vi "Main.vi"() -> ()   [LabVIEW 2017]
uses:
  <vilib>/rvi/Analysis/control/PID/Typedef/niFpgaPID_PIGains.ctl
  modulationConfig.ctl
  FPGA/contState.ctl
  <vilib>/NI/PowerElectronicsControl/ScaleAndLimit/Interface/Configuration.ctl
  <vilib>/NI/PowerElectronicsControl/BufferLogging/BufferConfig.ctl
  TuningParameters.ctl
  <instrlib>/_niInstr/FIFO Register Bus/v1/Host/niInstr FIFO Register Bus v1 Host.lvclass
  C:/Program Files (x86)/National Instruments/LabVIEW 2017/instr.lib/_niInstr/Instruction Framework/v1/Host/Instruction Target/niInstr Instruction Target v1 Host.lvclass
  <vilib>/FPGAPlugInAG/sbRIO-9607/niLvFpga_Open_sbRIO-9607.vi
  <vilib>/rvi/interface/common/dynamic/niFpgaDynamicAddResources.vi
  <vilib>/FPGAPlugInAG/Dynamic/niLvFpga_Reset_Dynamic.vi
  <vilib>/FPGAPlugInAG/Dynamic/niLvFpga_Run_Dynamic.vi
  <vilib>/Utility/error.llb/Error Cluster From Error Code.vi
  <vilib>/RVI Host/nirviSupport.llb/nirviErrorClusterFromErrorCode.vi
  <vilib>/rvi/errors/niLvFpgaAdjustHostInterfaceError.vi
  <vilib>/NI/PowerElectronicsControl/WaveformAcq/RT/ReadInterleaved.vi
  <vilib>/FPGAPlugInAG/Dynamic/niLvFpga_Close_Dynamic.vi
  <vilib>/rvi/interface/nirviOpenFPGA/nirviOpenFPGA.xnode
  FPGA Bitfiles/BuckBoost_FPGATarget_Firmware_5T++5BilX3c.lvbitx
  FPGA/Firmware.vi
  <vilib>/rvi/interface/nirviMethod/nirviMethod.xnode
  <vilib>/rvi/interface/nirviReadWriteControl/nirviReadWriteControl.xnode
  <vilib>/rvi/interface/nirviCloseFPGA/nirviCloseFPGA.xnode
  <vilib>/NI/PowerElectronicsControl/ScaleAndLimit/Interface/ScaleAndLimitInterface.lvlib
  <instrlib>/_niInstr/Instruction Framework/v1/Host/Subsystem Map/niInstr Subsystem Map v1 Host.lvclass
  <vilib>/NI/PowerElectronicsControl/WaveformAcq/RT/WaveformTask.lvclass
  <vilib>/NI/PowerElectronicsControl/BufferLogging/BufferLogging.lvlib
  <vilib>/rvi/interface/nirviMethod/StockFPGA_InlinedMethodWaitForSingleIRQ.vi
  <vilib>/FPGAPlugInAG/Dynamic/niLvFpga_WaitOnIrq_Dynamic.vi
  <vilib>/rvi/interface/Simulation/niFpgaSimulationCallBeginRW.vi
  <vilib>/FPGAPlugInAG/Dynamic/niLvFpga_AcknowledgeIrq_Dynamic.vi
  NiFpgaLv.dll
  BuckBoostInterface.lvlib
  FPGA/BuckBoost.lvlib
panel:
  in  "Tab Control":enum32{"Monitoring", "BuckBoost"}(tab)=enum."BuckBoost"
  out "SimultaneousAI":sgl[](array[numeric])=[-0.17586, 0.33218002, -0.12701, 12.40282, 40.089428, 0.0, 0.0, 0.0, -0.0, 0.0, 0.0, 0.0, 0.0, 0.0, 0.0, 0.0]
  out "snapshot":waveform(sgl)[](graph)=[{"t0"=timestamp(0 s since 1904-01-01), "dt"=1e-05, "Y"=array[10000 elements]}, {"t0"=timestamp(0 s since 1904-01-01), "dt"=1e-05, "Y"=array[10000 elements]}, {"t0"=timestamp(0 s since 1904-01-01), "dt"=1e-05, "Y"=array[10000 elements]}, {"t0"=timestamp(0 s since 1904-01-01), "dt"=1e-05, "Y"=array[10000 elements]}, {"t0"=timestamp(0 s since 1904-01-01), "dt"=1e-05, "Y"=array[10000 elements]}, {"t0"=timestamp(0 s since 1904-01-01), "dt"=1e-05, "Y"=array[10000 elements]}, {"t0"=timestamp(0 s since 1904-01-01), "dt"=1e-05, "Y"=array[10000 elements]}, {"t0"=timestamp(0 s since 1904-01-01), "dt"=1e-05, "Y"=array[10000 elements]}, {"t0"=timestamp(0 s since 1904-01-01), "dt"=1e-05, "Y"=array[10000 elements]}, {"t0"=timestamp(0 s since 1904-01-01), "dt"=1e-05, "Y"=array[10000 elements]}, {"t0"=timestamp(0 s since 1904-01-01), "dt"=1e-05, "Y"=array[10000 elements]}, {"t0"=timestamp(0 s since 1904-01-01), "dt"=1e-05, "Y"=array[10000 elements]}, {"t0"=timestamp(0 s since 1904-01-01), "dt"=1e-05, "Y"=array[10000 elements]}, {"t0"=timestamp(0 s since 1904-01-01), "dt"=1e-05, "Y"=array[10000 elements]}, {"t0"=timestamp(0 s since 1904-01-01), "dt"=1e-05, "Y"=array[10000 elements]}, {"t0"=timestamp(0 s since 1904-01-01), "dt"=1e-05, "Y"=array[10000 elements]}, {"t0"=timestamp(0 s since 1904-01-01), "dt"=1e-05, "Y"=array[10000 elements]}, {"t0"=timestamp(0 s since 1904-01-01), "dt"=1e-05, "Y"=array[10000 elements]}]
  in  "Update Time (s)":dbl=2.0 caption="Time Target (s)" min=1.0
  in  "stop":bool
  in  "clearLimits":bool
  out "SimultaneousAILoopRate":u32=800
  out "Limits":string="Zero limits reached"
  in  "ManualTrigger":bool
  out "TotalCurrent":sgl
  out "Enabled":u8=7 format="%.0x"
  in  "I_setpt":sgl=10.0
  out "error":sgl[](array[numeric])=[0.17586, -0.33218002, 0.12701, 0.0]
  in  "Enable":bool=TRUE
  in  "pertAmp":sgl=1.0
  in  "pertFreq":sgl=10.0
  in  "controlFreq":sgl=50000.0
  in  "rampRate":sgl=0.0001
  in  "state":T1=enum."normal"
  in  "gains":T2={"proportional gain"=0.1, "integral gain"=1e-05} {"proportional gain" step=0.125}
  in  "modulationConfig":T3={"SwitchingSpeed"=5000.0, "Deadband"=1e-07, "modulationRate"=40000000.0}
  in  "manualInput":sgl
  in  "UpdateConfig":bool
  out "actualBuckBoostRate":u32=800
  # "CAREFUL"
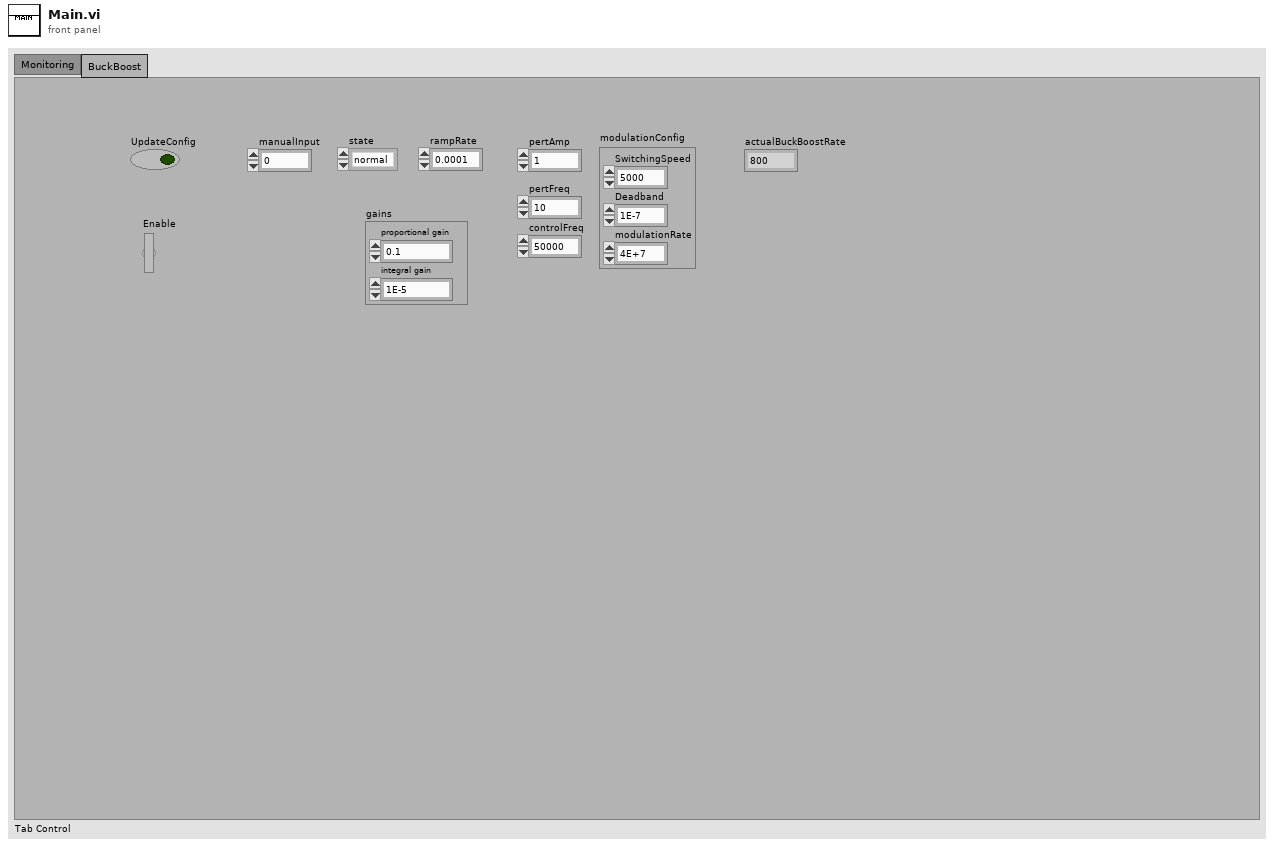
[diagram p1: front panel]
types:
  T1 = typedef "BuckBoost.lvlib/contState.ctl" = enum16{"disabled", "manual", "normal", "perturb"}
  T2 = typedef "niFpgaPID_PIGains.ctl" = cluster{"proportional gain":sgl, "integral gain":sgl}
  T3 = typedef "BuckBoostInterface.lvlib/modulationConfig.ctl" = cluster{"SwitchingSpeed":dbl, "Deadband":dbl, "modulationRate":dbl}
  T4 = typedef "BuckBoostInterface.lvlib/TuningParameters.ctl" = cluster{"gains":T2, "manualInput":sgl, "rampRate":sgl, "pertAmp":sgl, "pertFreq":sgl, "controlFreq":sgl, "state":T1}
  T5 = typedef "BufferLogging.lvlib/BufferConfig.ctl" = cluster{"Channels":string[], "pretriggerTime_sec":dbl, "posttriggerTime_sec":dbl, "BlockSizePerChannel":i32, "SampleRate_Hz":dbl, "decimation factor":i32, "logDirectory":string, "logPrefix":string, "max files":i32}
  T6 = typedef "ScaleAndLimitInterface.lvlib/Configuration.ctl" = cluster{"Name":string, "M":dbl, "B":i16, "HighLimit":dbl, "LowLimit":dbl, "LimitsEnabled":bool}
  T7 = typedef "BufferLogging.lvlib/Buffers.ctl" = cluster{"Channels":string[], "PosttriggerBuffer":refnum<queue>, "PretriggerBuffer":refnum<queue>, "BlockSizePerChannel":i32, " logging semaphore":T8, "Log refnum":refnum<k34>, "snapshotBuffer":refnum<data-value>, "logDirectory":path, "logPrefix":string, "decimation factor":i32, "max files":i32, "SampleRate":dbl}
  T8 = typedef "Semaphore RefNum" = refnum<k1>
  T9 = typedef "BuckBoostInterface.lvlib/Interface.ctl" = cluster{"instruction target":refnum<class "niInstr Instruction Target v1 Host.lvclass">, "BuckBoostContext":refnum<class "niInstr Instruction Framework Context v1 Host.lvclass">}
  T10 = typedef "ScaleAndLimitInterface.lvlib/Interface.ctl" = cluster{"instruction target":refnum<class "niInstr Instruction Target v1 Host.lvclass">, "ScalingAndLimitsContext":refnum<class "niInstr Instruction Framework Context v1 Host.lvclass">, "Configuration":T6[]}
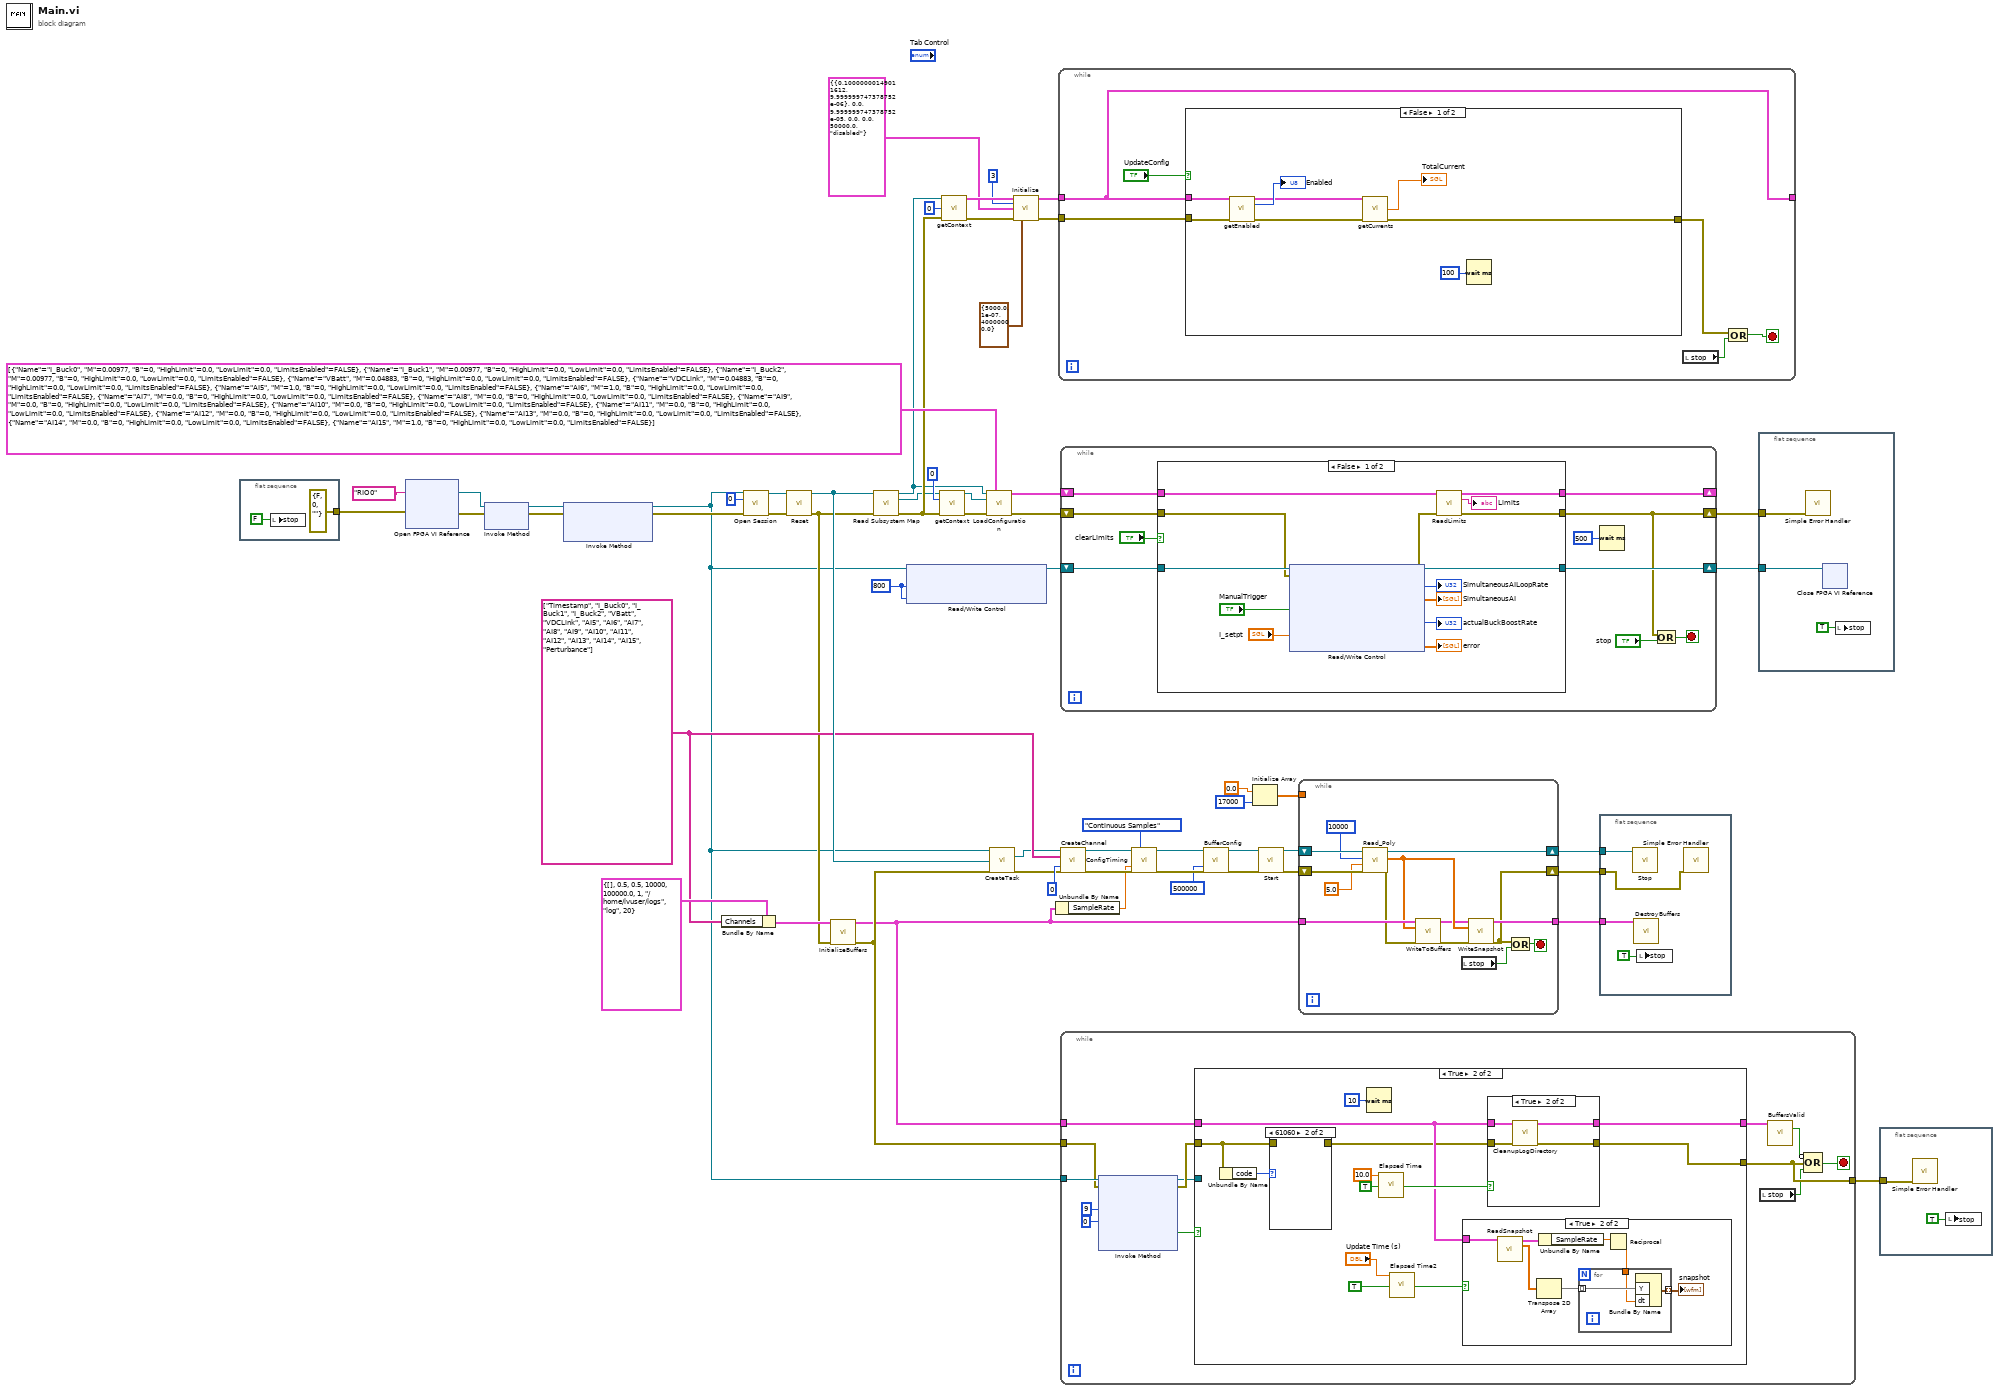
[diagram p0: block diagram]
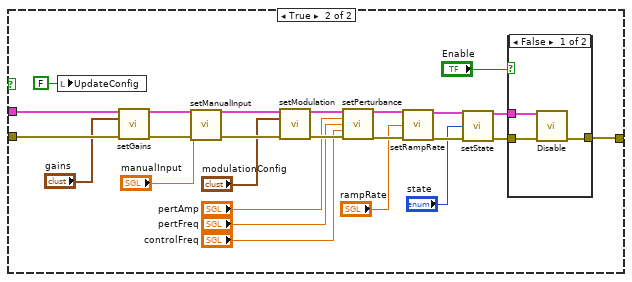
[diagram p2: hidden frame]
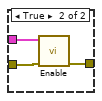
[diagram p3: hidden frame]
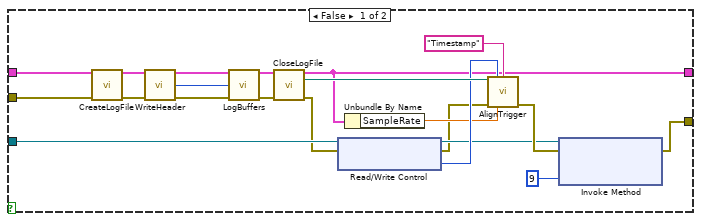
[diagram p4: hidden frame]
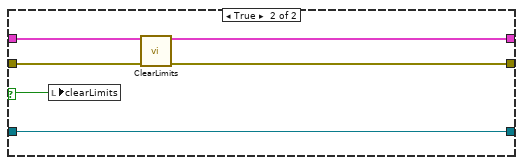
[diagram p8: hidden frame]
diagram:
  w13 = u32 800 ("desiredBuckBoostRate")
  w49 = string[] ["Timestamp", "I_Buck0", "I_Buck1", "I_Buck2", "VBatt", "VDCLink", "AI5", "AI6", "AI7", "AI8", "AI9", "AI10", "AI11", "AI12", "AI13", "AI14", "AI15", "Perturbance"] ("Chan Name Array")
  n1 = flat-sequence {
    tunnel: [errorcluster {"status"=FALSE, "code"=0, "source"=""} ("error in")] -> w46
    frame #0 {
      n2 = local write "stop"(FALSE ("stop")) -> ()
    }
  }
  n3 = xnode "Open FPGA VI Reference"("error in"=w46, "resource name"=tag "RIO0") -> ("FPGA VI Reference Out"=w6:refnum<k20>, "error out"=w5:errorcluster)
  n4 = xnode "Invoke Method"("FPGA VI Reference In"=w6, "error in"=w5) -> ("FPGA VI Reference Out"=w4:refnum<k20>, "error out"=w3:errorcluster)
  n5 = xnode "Invoke Method"("FPGA VI Reference In"=w4, "error in"=w3) -> ("FPGA VI Reference Out"=w1:refnum<k20>, "error out"=w2:errorcluster)  [unwired: 1 in]
  n6 = Bundle By Name(cluster=T5 {"Channels"=[], "pretriggerTime_sec"=0.5, "posttriggerTime_sec"=0.5, "BlockSizePerChannel"=10000, "SampleRate_Hz"=100000.0, "decimation factor"=1, "logDirectory"="/home/lvuser/logs", "logPrefix"="log", "max files"=20} ("BufferConfig"), "Channels"=w49) -> (w48:T5)
  n7 = call <instrlib>:"Open Session.vi"("fpga ref"=w1, "bus instance"=u32 0, "error in"=w2) -> ("session out"=w53:refnum<class "niInstr FIFO Register Bus v1 Host.lvclass">, "error out"=w54:errorcluster)  [unwired: 11 in]
  n8 = call-dynamic "Reset.vi"("session in"=w53, "error in"=w54) -> ("session out"=w51:refnum<class "niInstr FIFO Register Bus v1 Host.lvclass">, "error out"=w47:errorcluster)  [unwired: 12 in]
  n9 = call <vilib>:"InitializeBuffers.vi"("BufferConfig"=w48, "error in (no error)"=w47) -> ("Buffers"=w43:T7, "error out"=w44:errorcluster)  [unwired: 12 in]
  n10 = call <instrlib>:"Read Subsystem Map.vi"("instruction target in"=w51, "error in"=w47) -> ("instruction target out"=w9:refnum<class "niInstr FIFO Register Bus v1 Host.lvclass">, "subsystem map"=w8:refnum<class "niInstr Subsystem Map v1 Host.lvclass">, "error out"=w11:errorcluster)  [unwired: 11 in]
  n11 = xnode "Read/Write Control"("FPGA VI Reference In"=w1, "desiredBuckBoostRate"=w13, "desiredSimultaneousAILoopRate"=w13) -> ("FPGA VI Reference Out"=w14:refnum<k20>)  [unwired: 1 in, 1 out]
  n12 = call <vilib>:"getContext.vi"("subsystemMap"=w8, "instance"=u8 0, "error in"=w11) -> ("ScalingAndLimitsContext"=w10:refnum<class "niInstr Instruction Framework Context v1 Host.lvclass">, "error out"=w60:errorcluster)  [unwired: 11 in]
  n13 = call <vilib>:"getContext.vi"("instruction target in"=w9, "instance"=u8 0, "error in"=w11) -> ("Interface"=w20:T9, "error out"=w19:errorcluster)  [unwired: 11 in]
  n14 = call <vilib>:"LoadConfiguration.vi"("instruction target in"=w9, "Configuration"=T6[] [{"Name"="I_Buck0", "M"=0.00977, "B"=0, "HighLimit"=0.0, "LowLimit"=0.0, "LimitsEnabled"=FALSE}, {"Name"="I_Buck1", "M"=0.00977, "B"=0, "HighLimit"=0.0, "LowLimit"=0.0, "LimitsEnabled"=FALSE}, {"Name"="I_Buck2", "M"=0.00977, "B"=0, "HighLimit"=0.0, "LowLimit"=0.0, "LimitsEnabled"=FALSE}, {"Name"="VBatt", "M"=0.04883, "B"=0, "HighLimit"=0.0, "LowLimit"=0.0, "LimitsEnabled"=FALSE}, {"Name"="VDCLink", "M"=0.04883, "B"=0, "HighLimit"=0.0, "LowLimit"=0.0, "LimitsEnabled"=FALSE}, {"Name"="AI5", "M"=1.0, "B"=0, "HighLimit"=0.0, "LowLimit"=0.0, "LimitsEnabled"=FALSE}, {"Name"="AI6", "M"=1.0, "B"=0, "HighLimit"=0.0, "LowLimit"=0.0, "LimitsEnabled"=FALSE}, {"Name"="AI7", "M"=0.0, "B"=0, "HighLimit"=0.0, "LowLimit"=0.0, "LimitsEnabled"=FALSE}, {"Name"="AI8", "M"=0.0, "B"=0, "HighLimit"=0.0, "LowLimit"=0.0, "LimitsEnabled"=FALSE}, {"Name"="AI9", "M"=0.0, "B"=0, "HighLimit"=0.0, "LowLimit"=0.0, "LimitsEnabled"=FALSE}, {"Name"="AI10", "M"=0.0, "B"=0, "HighLimit"=0.0, "LowLimit"=0.0, "LimitsEnabled"=FALSE}, {"Name"="AI11", "M"=0.0, "B"=0, "HighLimit"=0.0, "LowLimit"=0.0, "LimitsEnabled"=FALSE}, {"Name"="AI12", "M"=0.0, "B"=0, "HighLimit"=0.0, "LowLimit"=0.0, "LimitsEnabled"=FALSE}, {"Name"="AI13", "M"=0.0, "B"=0, "HighLimit"=0.0, "LowLimit"=0.0, "LimitsEnabled"=FALSE}, {"Name"="AI14", "M"=0.0, "B"=0, "HighLimit"=0.0, "LowLimit"=0.0, "LimitsEnabled"=FALSE}, {"Name"="AI15", "M"=1.0, "B"=0, "HighLimit"=0.0, "LowLimit"=0.0, "LimitsEnabled"=FALSE}], "ScalingAndLimitsContext"=w10, "error in (no error)"=w60) -> ("Interface"=w57:T10, "error out"=w56:errorcluster)  [unwired: 10 in]
  n15 = call <vilib>:"CreateTask.vi"("FPGA Ref in"=w1, "session in"=w51, "error in"=w44) -> ("Task out"=w30:refnum<class "WaveformTask.lvclass">, "error out"=w29:errorcluster)  [unwired: 9 in, 2 out]
  n16 = call "Initialize.vi"("Interface in"=w20, "numOfInterleaves"=u8 3, "TuningParameters"=T4 {"gains"={"proportional gain"=0.1, "integral gain"=1e-05}, "manualInput"=0.0, "rampRate"=0.0001, "pertAmp"=0.0, "pertFreq"=0.0, "controlFreq"=50000.0, "state"=enum."disabled"}, "error in"=w19, "modulationConfig"=T3 {"SwitchingSpeed"=5000.0, "Deadband"=1e-07, "modulationRate"=40000000.0}) -> ("Interface out"=w16:T9, "error out"=w15:errorcluster)  [unwired: 9 in]
  n17 = Unbundle By Name(w43) -> ("SampleRate"=w26:dbl)
  n18 = while {
    tunnel: w16 -> [w67]
    tunnel: w15 -> [w68]
    tunnel: [w67] -> _
    stop <- w65 stop-if-true
    n19 = case shown="False" "UpdateConfig" {
      tunnel: w68 -> [w72 w100]
      tunnel: w67 -> [w73 w101]
      tunnel: [w69 w77] -> w64
      frame False {
        n20 = call "getEnabled.vi"("Interface in"=w73, "error in (no error)"=w72) -> ("Interface out"=w70:T9, "Enabled"=→"Enabled":u8, "error out"=w71:errorcluster)  [unwired: 11 in]
        n21 = call "getCurrents.vi"("Interface in"=w70, "error in (no error)"=w71) -> ("TotalCurrent"=→"TotalCurrent":sgl, "error out"=w69:errorcluster)  [unwired: 10 in, 2 out]
        n22 = Wait (ms)(milliseconds to wait=u32 100) -> ()  [unwired: 1 out]
      }
      frame True {
        n23 = local write "UpdateConfig"(FALSE ("UpdateConfig")) -> ()
        n24 = call "setGains.vi"("Interface in"=w101, "gains"="gains", "error in (no error)"=w100) -> ("Interface out"=w98:T9, "error out"=w99:errorcluster)  [unwired: 11 in]
        n25 = call "setManualInput.vi"("Interface in"=w98, "manualInput"="manualInput", "error in (no error)"=w99) -> ("Interface out"=w97:T9, "error out"=w96:errorcluster)  [unwired: 11 in]
        n26 = call "setModulation.vi"("Interface in"=w97, "modulationConfig"="modulationConfig", "error in (no error)"=w96) -> ("Interface out"=w94:T9, "error out"=w95:errorcluster)  [unwired: 11 in]
        n27 = call "setPerturbance.vi"("Interface in"=w94, "pertAmp"="pertAmp", "pertFreq"="pertFreq", "controlFreq"="controlFreq", "error in (no error)"=w95) -> ("Interface out"=w93:T9, "error out"=w90:errorcluster)  [unwired: 9 in]
        n28 = call "setRampRate.vi"("Interface in"=w93, "rampRate"="rampRate", "error in (no error)"=w90) -> ("Interface out"=w92:T9, "error out"=w91:errorcluster)  [unwired: 11 in]
        n29 = call "setState.vi"("Interface in"=w92, "state"="state", "error in (no error)"=w91) -> ("Interface out"=w79:T9, "error out"=w78:errorcluster)  [unwired: 11 in]
        n30 = case shown="False" "Enable" {
          tunnel: w79 -> [w102 w107]
          tunnel: w78 -> [w104 w106]
          tunnel: [w103 w105] -> w77
          frame False {
            n31 = call "Disable.vi"("Interface in"=w102, "error in (no error)"=w104) -> ("error out"=w103:errorcluster)  [unwired: 12 in, 1 out]
          }
          frame True {
            n32 = call "Enable.vi"("Interface in"=w107, "error in (no error)"=w106) -> ("error out"=w105:errorcluster)  [unwired: 12 in, 1 out]
          }
        }
      }
    }
    n33 = local read "stop"() -> (w63:bool)
    n34 = Compound Arithmetic op=OR(w64, w63) -> (w65:bool)
  }
  n35 = call <vilib>:"CreateChannel.vi"("task in"=w30, "Chan Name Array"=w49, "instance"=u8 0, "error in"=w29) -> ("Task out"=w31:refnum<class "WaveformTask.lvclass">, "error out"=w40:errorcluster)  [unwired: 10 in]
  n36 = while {
    tunnel: w44 -> [w112]
    tunnel: w43 -> [w120]
    tunnel: w1 -> [w116]
    tunnel: [w109] -> w42
    stop <- w118 stop-if-true
    n37 = xnode "Invoke Method"("FPGA VI Reference In"=w116, "error in"=w112, "IRQ Number(s)"=9, "Timeout (ms)"=0) -> ("FPGA VI Reference Out"=w110:refnum<k20>, "error out"=w111:errorcluster, "Timed Out"=w113:bool)  [unwired: 1 out]
    n38 = case shown="True" w113 {
      tunnel: w111 -> [w141 w144]
      tunnel: w120 -> [w140 w145]
      tunnel: [w125 w149] -> w119
      tunnel: [w131 w150] -> w109
      tunnel: w110 -> [w127 _]
      frame False {
        n39 = call <vilib>:"CreateLogFile.vi"("Buffers in"=w140, "error in (no error)"=w141) -> ("Buffers out"=w139:T7, "error out"=w138:errorcluster)  [unwired: 12 in]
        n40 = call <vilib>:"WriteHeader.vi"("Buffers in"=w139, "error in (no error)"=w138) -> ("Buffers out"=w137:T7, "numOfChannels"=w135:i32, "error out"=w136:errorcluster)  [unwired: 11 in]
        n41 = call <vilib>:"LogBuffers.vi"("Buffers in"=w137, "numOfChannels"=w135, "error in (no error)"=w136) -> ("Buffers out"=w134:T7, "error out"=w133:errorcluster)  [unwired: 11 in]
        n42 = call <vilib>:"CloseLogFile.vi"("Buffers in"=w134, "error in (no error)"=w133) -> ("Buffers out"=w125:T7, "log path out"=w130:path, "error out"=w123:errorcluster)  [unwired: 11 in]
        n43 = xnode "Read/Write Control"("FPGA VI Reference In"=w127, "error in"=w123) -> ("FPGA VI Reference Out"=w122:refnum<k20>, "error out"=w121:errorcluster, "TriggerTimestamp"=w126:i32)
        n44 = Unbundle By Name(w125) -> ("SampleRate"=w124:dbl)
        n45 = call <vilib>:"AlignTrigger.vi"("log path in"=w130, "triggerTimestamp"=w126, "alignmentChannel"="Timestamp", "error in (no error)"=w121, "AcqRate"=w124) -> ("error out"=w128:errorcluster)  [unwired: 9 in, 1 out]
        n46 = xnode "Invoke Method"("FPGA VI Reference In"=w122, "error in"=w128, "IRQ Number(s)"=9) -> ("error out"=w131:errorcluster)  [unwired: 1 out]
      }
      frame True {
        n47 = Unbundle By Name(w144) -> ("code"=w143:i32)
        n48 = case shown="61060" w143 {
          tunnel: w144 -> [w155 _]
          tunnel: [w155 _] -> w142
          frame 0, Default {
          }
          frame 61060 {
          }
        }
        n49 = Wait (ms)(milliseconds to wait=u32 10) -> ()  [unwired: 1 out]
        n50 = call "Elapsed Time"("Time Target (s)"=10.0, "Auto Reset"=TRUE) -> ("Time has Elapsed"=w151:bool)  [unwired: 10 in, 7 out]
        n51 = call "Elapsed Time2"("Time Target (s)"="Update Time (s)", "Auto Reset"=TRUE) -> ("Time has Elapsed"=w146:bool)  [unwired: 10 in, 7 out]
        n52 = case shown="True" w146 {
          tunnel: w145 -> [_ w156]
          frame False {
          }
          frame True {
            n53 = call <vilib>:"ReadSnapshot.vi"("Buffers in"=w156) -> ("Buffers out"=w159:T7, "snapshot"=w162:sgl[][])  [unwired: 12 in, 1 out]
            n54 = Transpose 2D Array(2D array=w162) -> (transposed array=w161:sgl[][])
            n55 = Unbundle By Name(w159) -> ("SampleRate"=w158:dbl)
            n56 = Reciprocal(x=w158) -> (1/x=w157:dbl)
            n57 = for {
              tunnel: w161 -> [w165] mode=indexing
              tunnel: [w164] -> w160 mode=indexing
              tunnel: w157 -> [w163]
              n58 = Bundle By Name("Y"=w165, "dt"=w163) -> (w164:waveform(sgl))  [unwired: 1 in]
            }
            "snapshot" <- w160
          }
        }
        n59 = case shown="True" w151 {
          tunnel: w142 -> [w167 w171]
          tunnel: [w167 w170] -> w150
          tunnel: w145 -> [w166 w169]
          tunnel: [w166 w168] -> w149
          frame False {
          }
          frame True {
            n60 = call <vilib>:"CleanupLogDirectory.vi"("BuffersIn"=w169, "error in"=w171) -> ("BuffersOut"=w168:T7, "error out"=w170:errorcluster)  [unwired: 12 in]
          }
        }
      }
    }
    n61 = local read "stop"() -> (w108:bool)
    n62 = call <vilib>:"BuffersValid.vi"("Buffers in"=w119) -> ("valid"=w117:bool)  [unwired: 13 in, 1 out]
    n63 = Compound Arithmetic op=OR(invert w117, w109, w108) -> (w118:bool)
  }
  n64 = while {
    shift-right: [w175] -> _
    shift-left: w57 -> [w181]
    shift-right: [w173] -> w45
    shift-left: w56 -> [w180]
    shift-right: [w176] -> w55
    shift-left: w14 -> [w177]
    stop <- w174 stop-if-true
    n65 = case shown="False" "clearLimits" {
      selector: "clearLimits" -> [_ w196]
      tunnel: w181 -> [w192 w201]
      tunnel: w180 -> [w194 w200]
      tunnel: [w191 w199] -> w175
      tunnel: [w190 w198] -> w173
      tunnel: w177 -> [w195 w197]
      tunnel: [w193 w197] -> w176
      frame False {
        n66 = xnode "Read/Write Control"("FPGA VI Reference In"=w195, "error in"=w194, "ManualTrigger"="ManualTrigger", "I_setpt"="I_setpt") -> ("FPGA VI Reference Out"=w193:refnum<k20>, "error out"=w188:errorcluster, "actualSimultaneousAILoopRate"=→"SimultaneousAILoopRate":u32, "Simultaneous_AI"=→"SimultaneousAI":sgl[], "actualBuckBoostRate"=→"actualBuckBoostRate":u32, "errors"=→"error":sgl[])
        n67 = call <vilib>:"ReadLimits.vi"("Interface in"=w192, "error in (no error)"=w188) -> ("Interface out"=w191:T10, "Limits"=→"Limits":string, "error out"=w190:errorcluster)  [unwired: 11 in]
      }
      frame True {
        n68 = local write "clearLimits"(w196) -> ()
        n69 = call <vilib>:"ClearLimits.vi"("Interface in"=w201, "error in (no error)"=w200) -> ("Interface out"=w199:T10, "error out"=w198:errorcluster)  [unwired: 12 in]
      }
    }
    n70 = Wait (ms)(milliseconds to wait=u32 500) -> ()  [unwired: 1 out]
    n71 = Compound Arithmetic op=OR(w173, "stop") -> (w174:bool)
  }
  n72 = call <vilib>:"ConfigTiming.vi"("Task in"=w31, "Sample Mode"=enum16{"Finite Samples", "Continuous Samples"}."Continuous Samples", "Sample Rate"=w26, "error in (no error)"=w40) -> ("Task out"=w38:refnum<class "WaveformTask.lvclass">, "error out"=w37:errorcluster)  [unwired: 9 in, 1 out]
  n73 = call <vilib>:"BufferConfig.vi"("WaveformTask in"=w38, "Buffer Size [Samps per Chan]"=500000, "error in (no error)"=w37) -> ("WaveformTask out"=w35:refnum<class "WaveformTask.lvclass">, "error out"=w34:errorcluster)  [unwired: 10 in, 1 out]
  n74 = Initialize Array(0.0 ("element"), 17000 ("dimension size")) -> (w22:dbl[])
  n75 = call <vilib>:"Start.vi"("WaveformTask in"=w35, "error in (no error)"=w34) -> ("WaveformTask out"=w33:refnum<class "WaveformTask.lvclass">, "error out"=w32:errorcluster)  [unwired: 12 in]
  n76 = while {
    shift-right: [w207] -> w25
    shift-left: w32 -> [w214]
    shift-right: [w213] -> w28
    shift-left: w33 -> [w215]
    tunnel: w43 -> [w212]
    tunnel: [w210] -> w27
    tunnel: w22 -> [_]
    stop <- w206 stop-if-true
    n77 = call-poly <vilib>:"Read_Poly.vi"("error in"=w214, "Timeout (s)"=5.0, "Samps Read per Chan"=10000, "Task in"=w215) -> ("error out"=w202:errorcluster, "Data"=w211:sgl[], "Task out"=w213:refnum<class "WaveformTask.lvclass">)  [unwired: 4 in, 1 out]
    n78 = call <vilib>:"WriteToBuffers.vi"("Buffers in"=w212, "Data"=w211, "error in (no error)"=w202) -> ("Buffers out"=w208:T7, "error out"=w209:errorcluster)  [unwired: 11 in]
    n79 = local read "stop"() -> (w205:bool)
    n80 = call <vilib>:"WriteSnapshot.vi"("Buffers in"=w208, "Snapshot"=w211, "error in (no error)"=w209) -> ("Buffers out"=w210:T7, "error out"=w207:errorcluster)  [unwired: 11 in]
    n81 = Compound Arithmetic op=OR(w207, w205) -> (w206:bool)
  }
  n82 = flat-sequence {
    tunnel: w28 -> [w219]
    tunnel: w27 -> [w218]
    tunnel: w25 -> [w216]
    frame #0 {
      n83 = call <vilib>:"Stop.vi"("WaveformTask in"=w219) -> ()  [unwired: 9 in, 2 out]
      n84 = call <vilib>:"DestroyBuffers.vi"("Buffers"=w218) -> ()  [unwired: 14 in, 1 out]
      n85 = local write "stop"(TRUE ("stop")) -> ()
      n86 = call <vilib>:"Simple Error Handler.vi"("error in (no error)"=w216) -> ()  [unwired: 4 in, 5 out]
    }
  }
  n87 = flat-sequence {
    tunnel: w55 -> [w222]
    tunnel: w45 -> [w220]
    frame #0 {
      n88 = call <vilib>:"Simple Error Handler.vi"("error in (no error)"=w220) -> ()  [unwired: 4 in, 5 out]
      n89 = xnode "Close FPGA VI Reference"("FPGA VI Reference In"=w222) -> ()  [unwired: 1 in, 1 out]
      n90 = local write "stop"(TRUE ("stop")) -> ()
    }
  }
  n91 = flat-sequence {
    tunnel: w42 -> [w223]
    frame #0 {
      n92 = call <vilib>:"Simple Error Handler.vi"("error in (no error)"=w223) -> ()  [unwired: 4 in, 5 out]
      n93 = local write "stop"(TRUE ("stop")) -> ()
    }
  }
